vi "Handle Last Ack Core.vi"(4 "error in (no error)":errorcluster, 6 "Last Ack":refnum<class "Last Ack.lvclass">, 7 "Coffee Shop in":refnum<class "Coffee Shop.lvclass">) -> (0 "error out":errorcluster, 3 "Coffee Shop out":refnum<class "Coffee Shop.lvclass">)   [LabVIEW 2023, in "Coffee Shop.lvlib" / "Coffee Shop.lvclass"]
doc: "(<B>Filename</B>: Actor Framework.lvlib:Actor.lvclass:Handle Last Ack Core.vi)\n\nDefines how the caller actor responds to the Last Ack message from a nested actor. The Last Ack message is the final message a nested actor sends to its caller before it shuts down. The message contains information about the final state of the nested actor.\n\nBy default, this method does nothing except return any error the nested actor sent. A descendant class may override this method to define behavior."
uses:
  Coffee Shop.lvclass
  <vilib>/ActorFramework/LastAck/Last Ack.lvclass
  <vilib>/ActorFramework/LastAck/Last Ack.lvclass/Last Ack.ctl
  <vilib>/ActorFramework/Actor/Actor.lvclass/Actor.ctl
  <vilib>/ActorFramework/Message Enqueuer/Message Enqueuer.lvclass/Message Enqueuer.ctl
  Coffee Shop.lvclass/Coffee Shop.ctl
  <vilib>/ActorFramework/Message Enqueuer/Init from Existing Queue.vi
  <vilib>/ActorFramework/Message Enqueuer/Message Enqueuer.lvclass
  <vilib>/ActorFramework/Actor/Actor.lvclass
  Entity Table/Entity Table.lvclass
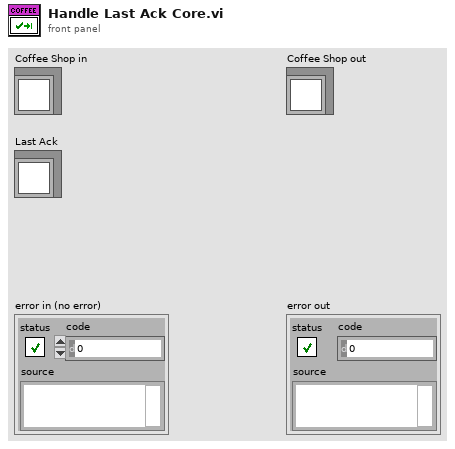
[diagram p1: front panel]
types:
  T1 = typedef "Coffee Shop.lvlib/Coffee Shop.lvclass/Entity Types.ctl" = enum16{"Customer", "Cashier", "Barista"}
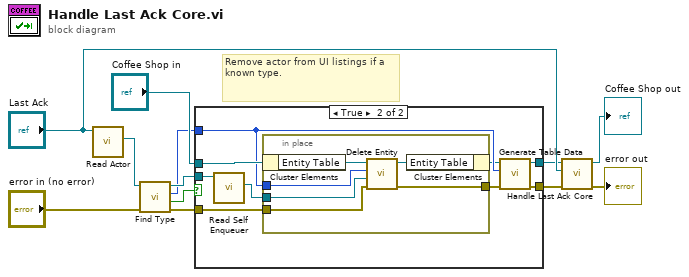
[diagram p0: block diagram]
diagram:
  # "Remove actor from UI listings if a known type."
  n1 = call <vilib>:"Read Actor.vi"("Last Ack"="Last Ack") -> ("Actor"=w9:refnum<class "Actor.lvclass">)  [unwired: 10 in]
  n2 = call "Find Type.vi"("error in"="error in (no error)", "Actor In"=w9) -> ("error out"=w6:errorcluster, "Type Found?"=w5:bool, "Entity Type"=w4:T1, "Actor Out"=w8:refnum<class "Actor.lvclass">)  [unwired: 6 in]
  n3 = case shown="True" w5 {
    tunnel: w8 -> [_ w23]
    tunnel: "Coffee Shop in" -> [w14 w21]
    tunnel: w6 -> [w13 w20]
    tunnel: w4 -> [_ w19]
    tunnel: [w14 w22] -> w3
    tunnel: [w13 w15] -> w1
    frame False {
    }
    frame True {
      n4 = call <vilib>:"Read Self Enqueuer.vi"("Actor"=w23) -> ("Self Enqueuer"=w16:refnum<class "Message Enqueuer.lvclass">)  [unwired: 10 in]
      n5 = in-place "In Place Element Structure" {
        in-place-border: w20 -> [w28]
        in-place-border: w19 -> [w27]
        in-place-border: [w25] -> w18
        in-place-border: w16 -> [w24]
        n6 = in-place-cluster #1 ("Unbundle / Bundle Elements")(w21) -> ("Entity Table"=w29:refnum<class "Entity Table.lvclass">)
        n7 = call "Delete Entity.vi"("error in (no error)"=w28, "enqueuer"=w24, "entity type"=w27, "entity table in"=w29) -> ("error out"=w25:errorcluster, "entity table out"=w26:refnum<class "Entity Table.lvclass">)  [unwired: 6 in]
        n8 = in-place-cluster #1 ("Unbundle / Bundle Elements")("Entity Table"=w26) -> (w17:refnum<class "Coffee Shop.lvclass">)
      }
      n9 = call-dynamic "Generate Table Data.vi"("error in (no error)"=w18, "Entity Type"=w19, "Coffee Shop in"=w17) -> ("error out"=w15:errorcluster, "Coffee Shop out"=w22:refnum<class "Coffee Shop.lvclass">)  [unwired: 7 in]
    }
  }
  n10 = call-parent "Handle Last Ack Core.vi"("error in (no error)"=w1, "Last Ack"="Last Ack", "Actor in"=w3) -> ("error out"=→"error out":errorcluster, "Actor out"=→"Coffee Shop out":refnum<class "Coffee Shop.lvclass">)  [unwired: 3 in]
